vi "test-pose3d.vi"(8 "error in (no error)":errorcluster) -> (0 "error out":errorcluster, 3 "All PASSED":bool)   [LabVIEW 2019]
uses:
  <vilib>/Rock Robotics/WPI/ThirdParty/JAS_Junk/TrajLib/VI/Pose3d_getTranslation3d.vi
  <vilib>/Rock Robotics/WPI/ThirdParty/JAS_Junk/TrajLib/VI/Transform3d_GetTranslation3d.vi
  <vilib>/Rock Robotics/WPI/ThirdParty/JAS_Junk/TrajLib/VI/Translation3d_Plus.vi
  <vilib>/Rock Robotics/WPI/ThirdParty/JAS_Junk/TrajLib/VI/Translation3d_RotateBy.vi
  <vilib>/Rock Robotics/WPI/ThirdParty/JAS_Junk/TrajLib/VI/Rotation3d_Plus.vi
  <vilib>/Rock Robotics/WPI/ThirdParty/JAS_Junk/TrajLib/Rotation2d_CreateAngle.vi
  <vilib>/Rock Robotics/WPI/ThirdParty/JAS_Junk/TrajLib/Translation2d_Create.vi
  <vilib>/Rock Robotics/WPI/ThirdParty/JAS_Junk/TrajLib/VI/Translation3d_ToTranslation2d.vi
  <vilib>/Rock Robotics/WPI/ThirdParty/JAS_Junk/TrajLib/VI/Rotation3d_ToRotation2d.vi
  <vilib>/Rock Robotics/WPI/ThirdParty/JAS_Junk/TrajLib/Pose2d_New_TRRO.vi
  <vilib>/Rock Robotics/WPI/ThirdParty/JAS_Junk/TrajLib/Translation2d_Equals.vi
  <vilib>/Rock Robotics/WPI/ThirdParty/JAS_Junk/TrajLib/Rotation2d_Equals.vi
  <vilib>/Rock Robotics/WPI/ThirdParty/JAS_Junk/TrajLib/VI/Rotation3d_Create_Default.vi
  <vilib>/Rock Robotics/WPI/ThirdParty/JAS_Junk/TrajLib/VI/Vector_Norm.vi
  <vilib>/Rock Robotics/WPI/ThirdParty/JAS_Junk/TrajLib/VecBuilder_ArrayBy1Fill.vi
  <vilib>/Rock Robotics/WPI/ThirdParty/JAS_Junk/TrajLib/VI/Translation3d_GetXYZ.vi
  <vilib>/Rock Robotics/WPI/ThirdParty/JAS_Junk/TrajLib/VI/Translation3d_Equals.vi
  <vilib>/Rock Robotics/WPI/ThirdParty/JAS_Junk/TrajLib/VI/Rotation3d_Equals.vi
  <vilib>/Rock Robotics/WPI/ThirdParty/JAS_Junk/TrajLib/VI/Transform3d_Create_Pose3dPose3d.vi
  <vilib>/Rock Robotics/WPI/ThirdParty/JAS_Junk/TrajLib/VI/Quaternion_Times.vi
  <vilib>/Rock Robotics/WPI/ThirdParty/JAS_Junk/TrajLib/VI/Quaternion_Inverse.vi
  <vilib>/Rock Robotics/WPI/ThirdParty/JAS_Junk/TrajLib/VI/Rotation3d_RotateBy.vi
  <vilib>/Rock Robotics/WPI/ThirdParty/JAS_Junk/TrajLib/Util_CalcDist.vi
  <vilib>/Rock Robotics/WPI/ThirdParty/JAS_Junk/TrajLib/VI/Quaternion_New_Default.vi
  <vilib>/Rock Robotics/WPI/ThirdParty/JAS_Junk/TrajLib/MatBuilder_Create.vi
  <vilib>/Rock Robotics/WPI/ThirdParty/JAS_Junk/TrajLib/VI/Quaternion_Equals.vi
  <vilib>/Rock Robotics/WPI/ThirdParty/JAS_Junk/TrajLib/VI/Translation3d_Minus.vi
  <vilib>/Rock Robotics/WPI/ThirdParty/JAS_Junk/TrajLib/VI/Rotation3d_UnaryMinus.vi
  <vilib>/Rock Robotics/WPI/ThirdParty/JAS_Junk/TrajLib/VI/Rotation3d_Minus.vi
  <vilib>/Rock Robotics/WPI/ThirdParty/JAS_Junk/TrajLib/VI/Quaternion_Get_Vect.vi
  <vilib>/Rock Robotics/WPI/ThirdParty/JAS_Junk/TrajLib/VI/Quaternion_Get_W.vi
  <vilib>/Rock Robotics/WPI/ThirdParty/JAS_Junk/TrajLib/VI/Quaternion_Normalize.vi
  <vilib>/Rock Robotics/WPI/ThirdParty/JAS_Junk/TrajLib/Trajectory_Library.lvlib
panel:
  out "Exp/Log \nTest Passed":bool
  # "Pose 3D test"
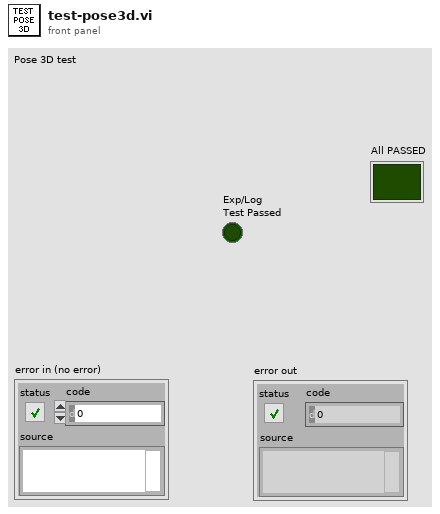
[diagram p1: front panel]
types:
  T1 = typedef "Trajectory_Library.lvlib/TRANSLATION3D.ctl" = cluster{"X":dbl, "Y":dbl, "Z":dbl}
  T2 = typedef "Trajectory_Library.lvlib/ROTATION3D.ctl" = cluster{"Q_quaternion":T3}
  T3 = typedef "Trajectory_Library.lvlib/QUATERNION.ctl" = cluster{"R":dbl, "V":dbl[]}
  T4 = typedef "Trajectory_Library.lvlib/POSE3D.ctl" = cluster{"Translation3d":T1, "Rotation3d":T2}
  T5 = typedef "Trajectory_Library.lvlib/TRANSFORM3D.ctl" = cluster{"TRANSLATION3D":T1, "ROTATION3D":T2, "XF":bool}
  T6 = typedef "Trajectory_Library.lvlib/POSE2D.ctl" = cluster{"TRANSLATION":T7, "ROTATION":T8}
  T7 = typedef "Trajectory_Library.lvlib/TRANSLATION2D.ctl" = cluster{"X":dbl, "Y":dbl}
  T8 = typedef "Trajectory_Library.lvlib/ROTATION2D.ctl" = cluster{"VALUE":dbl, "COS":dbl, "SIN":dbl}
  T9 = typedef "Trajectory_Library.lvlib/TWIST3D.ctl" = cluster{"dX":dbl, "dY":dbl, "dZ":dbl, "rX":dbl, "rY":dbl, "rZ":dbl}
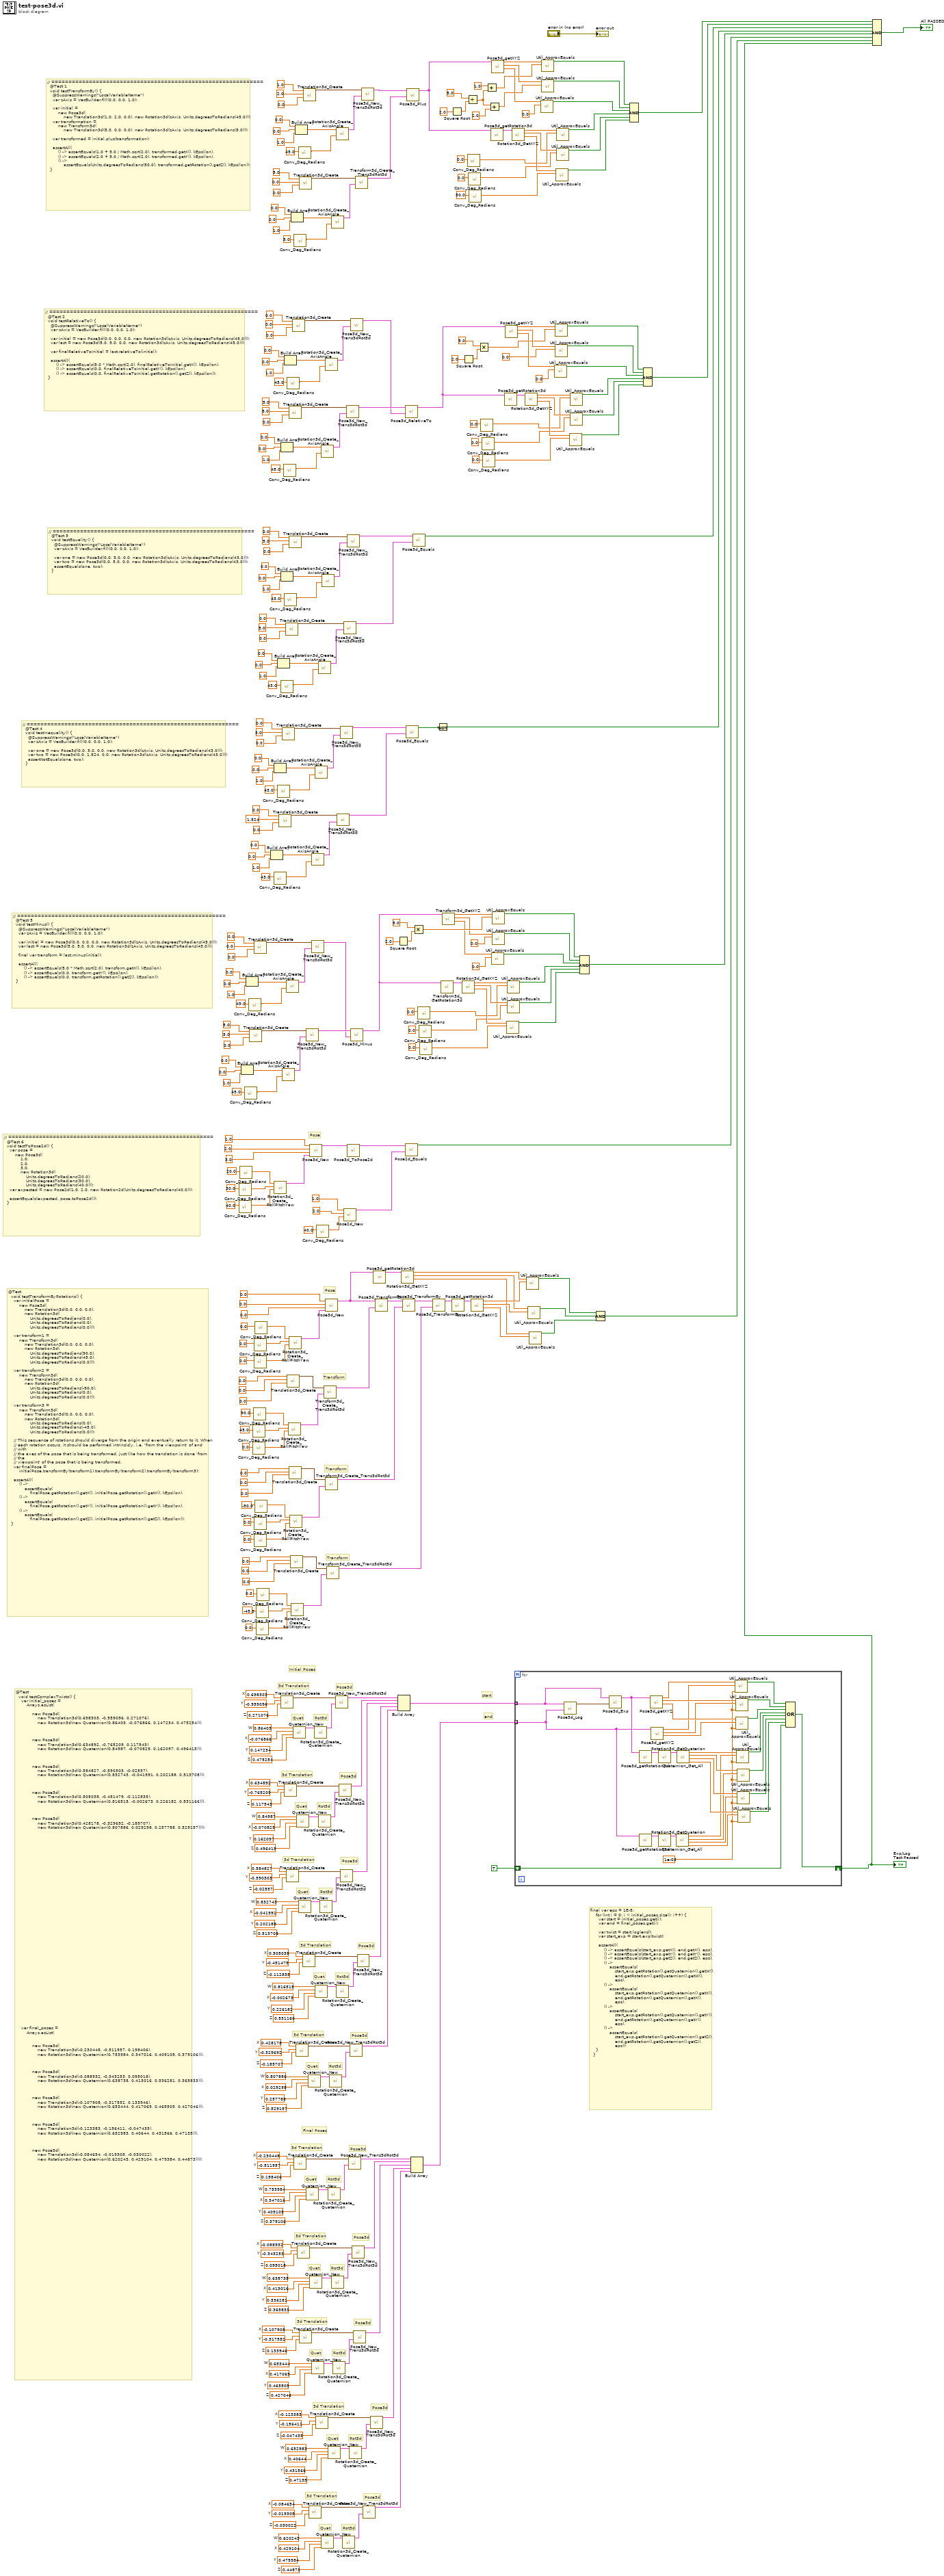
[diagram p0: block diagram]
diagram:
  w13 = 0.620243  # W
  w14 = 0.429104  # X
  w15 = 0.479384  # Y
  w16 = 0.44873  # Z
  w19 = -0.030022  # Z
  w18 = -0.084654  # X
  w17 = -0.019305  # Y
  w23 = 0.652983  # W
  w24 = 0.40644  # X
  w25 = 0.431566  # Y
  w26 = 0.47135  # Z
  w29 = -0.047435  # Z
  w28 = -0.123383  # X
  w27 = -0.156411  # Y
  w33 = 0.653444  # W
  w34 = 0.417069  # X
  w35 = 0.465505  # Y
  w36 = 0.427046  # Z
  w39 = 0.133946  # Z
  w38 = -0.107908  # X
  w37 = -0.317552  # Y
  w43 = 0.638738  # W
  w44 = 0.413016  # X
  w45 = 0.536281  # Y
  w46 = 0.365833  # Z
  w49 = 0.095018  # Z
  w48 = -0.088932  # X
  w47 = -0.343253  # Y
  w53 = 0.753984  # W
  w54 = 0.347016  # X
  w55 = 0.409105  # Y
  w56 = 0.379106  # Z
  w59 = 0.198406  # Z
  w58 = -0.230448  # X
  w57 = -0.511957  # Y
  w68 = 0.807886  # W
  w69 = 0.029298  # X
  w70 = 0.257788  # Y
  w71 = 0.529157  # Z
  w74 = -0.189707  # Z
  w73 = 0.428178  # X
  w72 = -0.329692  # Y
  w78 = 0.816515  # W
  w79 = -0.002673  # X
  w80 = 0.226182  # Y
  w81 = 0.531166  # Z
  w84 = -0.112835  # Z
  w83 = 0.505038  # X
  w82 = -0.451479  # Y
  w88 = 0.832743  # W
  w89 = -0.041991  # X
  w90 = 0.202188  # Y
  w91 = 0.513708  # Z
  w94 = -0.02557  # Z
  w93 = 0.584827  # X
  w92 = -0.590303  # Y
  w98 = 0.84987  # W
  w99 = -0.070829  # X
  w100 = 0.162097  # Y
  w101 = 0.496415  # Z
  w104 = 0.117543  # Z
  w103 = 0.634892  # X
  w102 = -0.765209  # Y
  w108 = 0.86403  # W
  w109 = -0.076866  # X
  w110 = 0.147234  # Y
  w111 = 0.475254  # Z
  w114 = 0.271076  # Z
  w113 = 0.698303  # X
  w112 = -0.959096  # Y
  # "end"
  # "start"
  # "final var eps = 1E-5;\n    for (int i = 0; i < initial_poses.size(); i++) {\n      var start = initial_poses.get(i);\n      var end = final_poses.get(i);\n\n      var twist = start.log(end);\n      var start_exp = start.exp(twist);\n\n      assertAll(\n          () -> assertEquals(start_exp.getX(), end.getX(), eps),\n          () -> assertEquals(start_exp.getY(), end.getY(), eps),\n          () -> assertEquals(start_exp.getZ(), end.getZ(), eps),\n          () ->\n              assertEquals(\n                  start_exp.getRotation().getQuaternion().getW(),\n                  end.getRotation().getQuaternion().getW(),\n                  eps),\n          () ->\n              assertEquals(\n                  start_exp.getRotation().getQuaternion().getX(),\n                  end.getRotation().getQuaternion().getX(),\n                  eps),\n          () ->\n              assertEquals(\n                  start_exp.getRotation().getQuaternion().getY(),\n                  end.getRotation().getQuaternion().getY(),\n                  eps),\n          () ->\n              assertEquals(\n                  start_exp.getRotation().getQuaternion().getZ(),\n                  end.getRotation().getQuaternion().getZ(),\n                  eps));\n    }\n  }"
  # "Rot3d"
  # "Pose3d"
  # "Quat"
  # "3d Translation"
  # "Rot3d"
  # "Pose3d"
  # "Quat"
  # "3d Translation"
  # "Rot3d"
  # "Pose3d"
  # "Quat"
  # "3d Translation"
  # "Rot3d"
  # "Pose3d"
  # "Quat"
  # "3d Translation"
  # "Final Poses"
  # "Rot3d"
  # "Pose3d"
  # "Quat"
  # "3d Translation"
  # "Rot3d"
  # "Pose3d"
  # "Quat"
  # "3d Translation"
  # "Rot3d"
  # "Pose3d"
  # "Quat"
  # "3d Translation"
  # "Rot3d"
  # "Pose3d"
  # "Quat"
  # "3d Translation"
  # "Rot3d"
  # "Pose3d"
  # "Quat"
  # "3d Translation"
  # "Initial Poses"
  # "Rot3d"
  # "Pose3d"
  # "Quat"
  # "3d Translation"
  # "@Test\n  void testComplexTwists() {\n    var initial_poses =\n        Arrays.asList(\n\n            new Pose3d(\n                new Translation3d(0.698303, -0.959096, 0.271076),\n                new Rotation3d(new Quaternion(0.86403, -0.076866, 0.147234, 0.475254))),\n\n\n\n            new Pose3d(\n                new Translation3d(0.634892, -0.765209, 0.117543),\n                new Rotation3d(new Quaternion(0.84987, -0.070829, 0.162097, 0.496415))),\n\n\n\n            new Pose3d(\n                new Translation3d(0.584827, -0.590303, -0.02557),\n                new Rotation3d(new Quaternion(0.832743, -0.041991, 0.202188, 0.513708))),\n\n\n\n            new Pose3d(\n                new Translation3d(0.505038, -0.451479, -0.112835),\n                new Rotation3d(new Quaternion(0.816515, -0.002673, 0.226182, 0.531166))),\n\n\n\n            new Pose3d(\n                new Translation3d(0.428178, -0.329692, -0.189707),\n                new Rotation3d(new Quaternion(0.807886, 0.029298, 0.257788, 0.529157))));\n\n\n\n\n\n\n\n\n\n\n\n\n\n\n\n\n\n\n\n\n\n\n\n\n\n\n\n\n\n\n\n\n\n\n\n\n\n\n\n\n\n\n\n\n\n    var final_poses =\n        Arrays.asList(\n\n\n            new Pose3d(\n                new Translation3d(-0.230448, -0.511957, 0.198406),\n                new Rotation3d(new Quaternion(0.753984, 0.347016, 0.409105, 0.379106))),\n\n\n\n            new Pose3d(\n                new Translation3d(-0.088932, -0.343253, 0.095018),\n                new Rotation3d(new Quaternion(0.638738, 0.413016, 0.536281, 0.365833))),\n\n\n\n            new Pose3d(\n                new Translation3d(-0.107908, -0.317552, 0.133946),\n                new Rotation3d(new Quaternion(0.653444, 0.417069, 0.465505, 0.427046))),\n\n\n\n            new Pose3d(\n                new Translation3d(-0.123383, -0.156411, -0.047435),\n                new Rotation3d(new Quaternion(0.652983, 0.40644, 0.431566, 0.47135))),\n\n\n\n            new Pose3d(\n                new Translation3d(-0.084654, -0.019305, -0.030022),\n                new Rotation3d(new Quaternion(0.620243, 0.429104, 0.479384, 0.44873))));"
  # "Transform"
  # "Transform"
  # "Transform"
  # "Pose"
  # "Pose"
  # "@Test\n  void testTransformByRotations() {\n    var initialPose =\n        new Pose3d(\n            new Translation3d(0.0, 0.0, 0.0),\n            new Rotation3d(\n                Units.degreesToRadians(0.0),\n                Units.degreesToRadians(0.0),\n                Units.degreesToRadians(0.0)));\n\n    var transform1 =\n        new Transform3d(\n            new Translation3d(0.0, 0.0, 0.0),\n            new Rotation3d(\n                Units.degreesToRadians(90.0),\n                Units.degreesToRadians(45.0),\n                Units.degreesToRadians(0.0)));\n\n    var transform2 =\n        new Transform3d(\n            new Translation3d(0.0, 0.0, 0.0),\n            new Rotation3d(\n                Units.degreesToRadians(-90.0),\n                Units.degreesToRadians(0.0),\n                Units.degreesToRadians(0.0)));\n\n    var transform3 =\n        new Transform3d(\n            new Translation3d(0.0, 0.0, 0.0),\n            new Rotation3d(\n                Units.degreesToRadians(0.0),\n                Units.degreesToRadians(-45.0),\n                Units.degreesToRadians(0.0)));\n\n    // This sequence of rotations should diverge from the origin and eventually return to it. When\n    // each rotation occurs, it should be performed intrinsicly, i.e. 'from the viewpoint' of and\n    // with\n    // the axes of the pose that is being transformed, just like how the translation is done 'from\n    // the\n    // viewpoint' of the pose that is being transformed.\n    var finalPose =\n        initialPose.transformBy(transform1).transformBy(transform2).transformBy(transform3);\n\n    assertAll(\n        () ->\n            assertEquals(\n                finalPose.getRotation().getX(), initialPose.getRotation().getX(), kEpsilon),\n        () ->\n            assertEquals(\n                finalPose.getRotation().getY(), initialPose.getRotation().getY(), kEpsilon),\n        () ->\n            assertEquals(\n                finalPose.getRotation().getZ(), initialPose.getRotation().getZ(), kEpsilon));\n  }"
  # "// ============================================================\n  @Test 6\n  void testToPose2d() {\n    var pose =\n        new Pose3d(\n            1.0,\n            2.0,\n            3.0,\n            new Rotation3d(\n                Units.degreesToRadians(20.0),\n                Units.degreesToRadians(30.0),\n                Units.degreesToRadians(40.0)));\n    var expected = new Pose2d(1.0, 2.0, new Rotation2d(Units.degreesToRadians(40.0)));\n\n    assertEquals(expected, pose.toPose2d());\n  }"
  # "// =============================================================\n  @Test 5\n  void testMinus() {\n    @SuppressWarnings(\"LocalVariableName\")\n    var zAxis = VecBuilder.fill(0.0, 0.0, 1.0);\n\n    var initial = new Pose3d(0.0, 0.0, 0.0, new Rotation3d(zAxis, Units.degreesToRadians(45.0)));\n    var last = new Pose3d(5.0, 5.0, 0.0, new Rotation3d(zAxis, Units.degreesToRadians(45.0)));\n\n    final var transform = last.minus(initial);\n\n    assertAll(\n        () -> assertEquals(5.0 * Math.sqrt(2.0), transform.getX(), kEpsilon),\n        () -> assertEquals(0.0, transform.getY(), kEpsilon),\n        () -> assertEquals(0.0, transform.getRotation().getZ(), kEpsilon));\n  }"
  # "// ==============================================================\n  @Test 4\n  void testInequality() {\n    @SuppressWarnings(\"LocalVariableName\")\n    var zAxis = VecBuilder.fill(0.0, 0.0, 1.0);\n\n    var one = new Pose3d(0.0, 5.0, 0.0, new Rotation3d(zAxis, Units.degreesToRadians(43.0)));\n    var two = new Pose3d(0.0, 1.524, 0.0, new Rotation3d(zAxis, Units.degreesToRadians(43.0)));\n    assertNotEquals(one, two);\n  }"
  # "// ===========================================================\n  @Test 3\n  void testEquality() {\n    @SuppressWarnings(\"LocalVariableName\")\n    var zAxis = VecBuilder.fill(0.0, 0.0, 1.0);\n\n    var one = new Pose3d(0.0, 5.0, 0.0, new Rotation3d(zAxis, Units.degreesToRadians(43.0)));\n    var two = new Pose3d(0.0, 5.0, 0.0, new Rotation3d(zAxis, Units.degreesToRadians(43.0)));\n    assertEquals(one, two);\n  }"
  # "// =============================================================\n  @Test 2\n  void testRelativeTo() {\n    @SuppressWarnings(\"LocalVariableName\")\n    var zAxis = VecBuilder.fill(0.0, 0.0, 1.0);\n\n    var initial = new Pose3d(0.0, 0.0, 0.0, new Rotation3d(zAxis, Units.degreesToRadians(45.0)));\n    var last = new Pose3d(5.0, 5.0, 0.0, new Rotation3d(zAxis, Units.degreesToRadians(45.0)));\n\n    var finalRelativeToInitial = last.relativeTo(initial);\n\n    assertAll(\n        () -> assertEquals(5.0 * Math.sqrt(2.0), finalRelativeToInitial.getX(), kEpsilon),\n        () -> assertEquals(0.0, finalRelativeToInitial.getY(), kEpsilon),\n        () -> assertEquals(0.0, finalRelativeToInitial.getRotation().getZ(), kEpsilon));\n  }"
  # "// ==============================================================\n  @Test 1\n  void testTransformBy() {\n    @SuppressWarnings(\"LocalVariableName\")\n    var zAxis = VecBuilder.fill(0.0, 0.0, 1.0);\n\n    var initial =\n        new Pose3d(\n            new Translation3d(1.0, 2.0, 0.0), new Rotation3d(zAxis, Units.degreesToRadians(45.0)));\n    var transformation =\n        new Transform3d(\n            new Translation3d(5.0, 0.0, 0.0), new Rotation3d(zAxis, Units.degreesToRadians(5.0)));\n\n    var transformed = initial.plus(transformation);\n\n    assertAll(\n        () -> assertEquals(1.0 + 5.0 / Math.sqrt(2.0), transformed.getX(), kEpsilon),\n        () -> assertEquals(2.0 + 5.0 / Math.sqrt(2.0), transformed.getY(), kEpsilon),\n        () ->\n            assertEquals(Units.degreesToRadians(50.0), transformed.getRotation().getZ(), kEpsilon));\n  }"
  n1 = call <vilib>:"Conv_Deg_Radians.vi"("Degress"=30.0) -> ("Radians"=w187:dbl)  [unwired: 10 in]
  n2 = call <vilib>:"Conv_Deg_Radians.vi"("Degress"=40.0) -> ("Radians"=w186:dbl)  [unwired: 10 in]
  n3 = call <vilib>:"Conv_Deg_Radians.vi"("Degress"=20.0) -> ("Radians"=w188:dbl)  [unwired: 10 in]
  n4 = Build Array(0.0 ("element"), 0.0 ("element"), 1.0 ("element")) -> (w234:dbl[])
  n5 = call <vilib>:"Conv_Deg_Radians.vi"("Degress"=45.0) -> ("Radians"=w232:dbl)  [unwired: 10 in]
  n6 = Build Array(0.0 ("element"), 0.0 ("element"), 1.0 ("element")) -> (w245:dbl[])
  n7 = call <vilib>:"Conv_Deg_Radians.vi"("Degress"=45.0) -> ("Radians"=w243:dbl)  [unwired: 10 in]
  n8 = call <vilib>:"Translation3d_Create.vi"("Z"=0.0, "Y"=5.0, "X"=5.0) -> ("TRANSLATION3D"=w225:T1)  [unwired: 8 in]
  n9 = call <vilib>:"Conv_Deg_Radians.vi"("Degress"=45.0) -> ("Radians"=w162:dbl)  [unwired: 10 in]
  n10 = call <vilib>:"Conv_Deg_Radians.vi"("Degress"=0.0) -> ("Radians"=w161:dbl)  [unwired: 10 in]
  n11 = call <vilib>:"Conv_Deg_Radians.vi"("Degress"=90.0) -> ("Radians"=w163:dbl)  [unwired: 10 in]
  n12 = call <vilib>:"Translation3d_Create.vi"("Z"=0.0, "Y"=0.0, "X"=0.0) -> ("TRANSLATION3D"=w236:T1)  [unwired: 8 in]
  n13 = call <vilib>:"Conv_Deg_Radians.vi"("Degress"=0.0) -> ("Radians"=w169:dbl)  [unwired: 10 in]
  n14 = call <vilib>:"Conv_Deg_Radians.vi"("Degress"=0.0) -> ("Radians"=w168:dbl)  [unwired: 10 in]
  n15 = call <vilib>:"Conv_Deg_Radians.vi"("Degress"=0.0) -> ("Radians"=w151:dbl)  [unwired: 10 in]
  n16 = call <vilib>:"Conv_Deg_Radians.vi"("Degress"=0.0) -> ("Radians"=w150:dbl)  [unwired: 10 in]
  n17 = call <vilib>:"Conv_Deg_Radians.vi"("Degress"=0.0) -> ("Radians"=w170:dbl)  [unwired: 10 in]
  n18 = call <vilib>:"Conv_Deg_Radians.vi"("Degress"=-90.0) -> ("Radians"=w152:dbl)  [unwired: 10 in]
  n19 = call <vilib>:"Conv_Deg_Radians.vi"("Degress"=-45.0) -> ("Radians"=w140:dbl)  [unwired: 10 in]
  n20 = call <vilib>:"Conv_Deg_Radians.vi"("Degress"=0.0) -> ("Radians"=w139:dbl)  [unwired: 10 in]
  n21 = call <vilib>:"Conv_Deg_Radians.vi"("Degress"=0.0) -> ("Radians"=w141:dbl)  [unwired: 10 in]
  n22 = Build Array(0.0 ("element"), 0.0 ("element"), 1.0 ("element")) -> (w260:dbl[])
  n23 = call <vilib>:"Conv_Deg_Radians.vi"("Degress"=43.0) -> ("Radians"=w258:dbl)  [unwired: 10 in]
  n24 = Build Array(0.0 ("element"), 0.0 ("element"), 1.0 ("element")) -> (w271:dbl[])
  n25 = call <vilib>:"Rotation3d_Create_RollPitchYaw.vi"("Yaw"=w186, "Pitch"=w187, "Roll"=w188) -> ("Rotation3d"=w185:T2)  [unwired: 8 in]
  n26 = Build Array(0.0 ("element"), 0.0 ("element"), 1.0 ("element")) -> (w285:dbl[])
  n27 = call <vilib>:"Conv_Deg_Radians.vi"("Degress"=43.0) -> ("Radians"=w269:dbl)  [unwired: 10 in]
  n28 = call <vilib>:"Translation3d_Create.vi"("Z"=0.0, "Y"=1.524, "X"=0.0) -> ("TRANSLATION3D"=w251:T1)  [unwired: 8 in]
  n29 = Build Array(0.0 ("element"), 0.0 ("element"), 1.0 ("element")) -> (w336:dbl[])
  n30 = call <vilib>:"Conv_Deg_Radians.vi"("Degress"=43.0) -> ("Radians"=w283:dbl)  [unwired: 10 in]
  n31 = Build Array(0.0 ("element"), 0.0 ("element"), 1.0 ("element")) -> (w296:dbl[])
  n32 = call <vilib>:"Translation3d_Create.vi"("Z"=w114, "Y"=w112, "X"=w113) -> ("TRANSLATION3D"=w107:T1)  [unwired: 8 in]
  n33 = call <vilib>:"Rotation3d_Create_AxisAngle.vi"("Angle"=w232, "Axis Vector"=w234) -> ("Rotation3d"=w224:T2)  [unwired: 9 in]
  n34 = call <vilib>:"Translation3d_Create.vi"("Z"=0.0, "Y"=5.0, "X"=0.0) -> ("TRANSLATION3D"=w262:T1)  [unwired: 8 in]
  n35 = call <vilib>:"Conv_Deg_Radians.vi"("Degress"=45.0) -> ("Radians"=w334:dbl)  [unwired: 10 in]
  n36 = Build Array(0.0 ("element"), 0.0 ("element"), 1.0 ("element")) -> (w347:dbl[])
  n37 = call <vilib>:"Conv_Deg_Radians.vi"("Degress"=43.0) -> ("Radians"=w294:dbl)  [unwired: 10 in]
  n38 = call <vilib>:"Translation3d_Create.vi"("Z"=w104, "Y"=w102, "X"=w103) -> ("TRANSLATION3D"=w97:T1)  [unwired: 8 in]
  n39 = call <vilib>:"Translation3d_Create.vi"("Z"=0.0, "Y"=5.0, "X"=0.0) -> ("TRANSLATION3D"=w276:T1)  [unwired: 8 in]
  n40 = call <vilib>:"Translation3d_Create.vi"("Z"=w94, "Y"=w92, "X"=w93) -> ("TRANSLATION3D"=w87:T1)  [unwired: 8 in]
  n41 = call <vilib>:"Rotation3d_Create_AxisAngle.vi"("Angle"=w243, "Axis Vector"=w245) -> ("Rotation3d"=w235:T2)  [unwired: 9 in]
  n42 = call <vilib>:"Conv_Deg_Radians.vi"("Degress"=45.0) -> ("Radians"=w345:dbl)  [unwired: 10 in]
  n43 = call <vilib>:"Translation3d_Create.vi"("Z"=0.0, "Y"=0.0, "X"=0.0) -> ("TRANSLATION3D"=w159:T1)  [unwired: 8 in]
  n44 = call <vilib>:"Rotation3d_Create_RollPitchYaw.vi"("Yaw"=w161, "Pitch"=w162, "Roll"=w163) -> ("Rotation3d"=w160:T2)  [unwired: 8 in]
  n45 = call <vilib>:"Translation3d_Create.vi"("Z"=0.0, "Y"=5.0, "X"=5.0) -> ("TRANSLATION3D"=w327:T1)  [unwired: 8 in]
  n46 = call <vilib>:"Translation3d_Create.vi"("Z"=0.0, "Y"=0.0, "X"=0.0) -> ("TRANSLATION3D"=w148:T1)  [unwired: 8 in]
  n47 = call <vilib>:"Translation3d_Create.vi"("Z"=0.0, "Y"=5.0, "X"=0.0) -> ("TRANSLATION3D"=w287:T1)  [unwired: 8 in]
  n48 = call <vilib>:"Rotation3d_Create_RollPitchYaw.vi"("Yaw"=w168, "Pitch"=w169, "Roll"=w170) -> ("Rotation3d"=w167:T2)  [unwired: 8 in]
  n49 = call <vilib>:"Rotation3d_Create_RollPitchYaw.vi"("Yaw"=w150, "Pitch"=w151, "Roll"=w152) -> ("Rotation3d"=w149:T2)  [unwired: 8 in]
  n50 = call <vilib>:"Translation3d_Create.vi"("Z"=0.0, "Y"=0.0, "X"=0.0) -> ("TRANSLATION3D"=w137:T1)  [unwired: 8 in]
  n51 = Build Array(0.0 ("element"), 0.0 ("element"), 1.0 ("element")) -> (w391:dbl[])
  n52 = call <vilib>:"Rotation3d_Create_RollPitchYaw.vi"("Yaw"=w139, "Pitch"=w140, "Roll"=w141) -> ("Rotation3d"=w138:T2)  [unwired: 8 in]
  n53 = call <vilib>:"Translation3d_Create.vi"("Z"=0.0, "Y"=0.0, "X"=0.0) -> ("TRANSLATION3D"=w338:T1)  [unwired: 8 in]
  n54 = call <vilib>:"Quaternion_New.vi"("Z"=w111, "Y"=w110, "X"=w109, "W"=w108) -> ("out Quaternion"=w106:T3)  [unwired: 7 in]
  n55 = call <vilib>:"Conv_Deg_Radians.vi"("Degress"=5.0) -> ("Radians"=w389:dbl)  [unwired: 10 in]
  n56 = call <vilib>:"Translation3d_Create.vi"("Z"=w59, "Y"=w57, "X"=w58) -> ("TRANSLATION3D"=w52:T1)  [unwired: 8 in]
  n57 = Build Array(0.0 ("element"), 0.0 ("element"), 1.0 ("element")) -> (w402:dbl[])
  n58 = call <vilib>:"Translation3d_Create.vi"("Z"=w74, "Y"=w72, "X"=w73) -> ("TRANSLATION3D"=w67:T1)  [unwired: 8 in]
  n59 = call <vilib>:"Quaternion_New.vi"("Z"=w101, "Y"=w100, "X"=w99, "W"=w98) -> ("out Quaternion"=w96:T3)  [unwired: 7 in]
  n60 = call <vilib>:"Translation3d_Create.vi"("Z"=w49, "Y"=w47, "X"=w48) -> ("TRANSLATION3D"=w42:T1)  [unwired: 8 in]
  n61 = call <vilib>:"Conv_Deg_Radians.vi"("Degress"=45.0) -> ("Radians"=w400:dbl)  [unwired: 10 in]
  n62 = call <vilib>:"Quaternion_New.vi"("Z"=w91, "Y"=w90, "X"=w89, "W"=w88) -> ("out Quaternion"=w86:T3)  [unwired: 7 in]
  n63 = call <vilib>:"Translation3d_Create.vi"("Z"=0.0, "Y"=0.0, "X"=5.0) -> ("TRANSLATION3D"=w382:T1)  [unwired: 8 in]
  n64 = call <vilib>:"Translation3d_Create.vi"("Z"=w39, "Y"=w37, "X"=w38) -> ("TRANSLATION3D"=w32:T1)  [unwired: 8 in]
  n65 = call <vilib>:"Translation3d_Create.vi"("Z"=w84, "Y"=w82, "X"=w83) -> ("TRANSLATION3D"=w77:T1)  [unwired: 8 in]
  n66 = call <vilib>:"Translation3d_Create.vi"("Z"=0.0, "Y"=2.0, "X"=1.0) -> ("TRANSLATION3D"=w393:T1)  [unwired: 8 in]
  n67 = call <vilib>:"Pose3d_New_Trans3dRot3d.vi"("Rotation3d"=w224, "Translation3d"=w225) -> ("outPose3d"=w197:T4)  [unwired: 9 in]
  n68 = call <vilib>:"Quaternion_New.vi"("Z"=w56, "Y"=w55, "X"=w54, "W"=w53) -> ("out Quaternion"=w51:T3)  [unwired: 7 in]
  n69 = call <vilib>:"Quaternion_New.vi"("Z"=w71, "Y"=w70, "X"=w69, "W"=w68) -> ("out Quaternion"=w66:T3)  [unwired: 7 in]
  n70 = call <vilib>:"Translation3d_Create.vi"("Z"=w19, "Y"=w17, "X"=w18) -> ("TRANSLATION3D"=w12:T1)  [unwired: 8 in]
  n71 = call <vilib>:"Pose3d_New.vi"("Rotation3d"=w185, "z"=3.0 ("Z"), "Y"=2.0, "X"=1.0) -> ("out Pose3d"=w184:T4)  [unwired: 7 in]
  n72 = call <vilib>:"Quaternion_New.vi"("Z"=w46, "Y"=w45, "X"=w44, "W"=w43) -> ("out Quaternion"=w41:T3)  [unwired: 7 in]
  n73 = call <vilib>:"Rotation3d_Create_AxisAngle.vi"("Angle"=w258, "Axis Vector"=w260) -> ("Rotation3d"=w250:T2)  [unwired: 9 in]
  n74 = call <vilib>:"Quaternion_New.vi"("Z"=w36, "Y"=w35, "X"=w34, "W"=w33) -> ("out Quaternion"=w31:T3)  [unwired: 7 in]
  n75 = call <vilib>:"Pose3d_New_Trans3dRot3d.vi"("Rotation3d"=w235, "Translation3d"=w236) -> ("outPose3d"=w196:T4)  [unwired: 9 in]
  n76 = call <vilib>:"Rotation3d_Create_Quaternion.vi"("Quaternion"=w106) -> ("Rotation3d"=w105:T2)  [unwired: 10 in]
  n77 = call <vilib>:"Rotation3d_Create_AxisAngle.vi"("Angle"=w269, "Axis Vector"=w271) -> ("Rotation3d"=w261:T2)  [unwired: 9 in]
  n78 = call <vilib>:"Quaternion_New.vi"("Z"=w81, "Y"=w80, "X"=w79, "W"=w78) -> ("out Quaternion"=w76:T3)  [unwired: 7 in]
  n79 = call <vilib>:"Translation3d_Create.vi"("Z"=w29, "Y"=w27, "X"=w28) -> ("TRANSLATION3D"=w22:T1)  [unwired: 8 in]
  n80 = call <vilib>:"Conv_Deg_Radians.vi"("Degress"=40.0) -> ("Radians"=w180:dbl)  [unwired: 10 in]
  n81 = call <vilib>:"Rotation3d_Create_AxisAngle.vi"("Angle"=w283, "Axis Vector"=w285) -> ("Rotation3d"=w275:T2)  [unwired: 9 in]
  n82 = call <vilib>:"Rotation3d_Create_Quaternion.vi"("Quaternion"=w96) -> ("Rotation3d"=w95:T2)  [unwired: 10 in]
  n83 = call <vilib>:"Rotation3d_Create_Quaternion.vi"("Quaternion"=w86) -> ("Rotation3d"=w85:T2)  [unwired: 10 in]
  n84 = call <vilib>:"Quaternion_New.vi"("Z"=w16, "Y"=w15, "X"=w14, "W"=w13) -> ("out Quaternion"=w11:T3)  [unwired: 7 in]
  n85 = call <vilib>:"Rotation3d_Create_AxisAngle.vi"("Angle"=w334, "Axis Vector"=w336) -> ("Rotation3d"=w326:T2)  [unwired: 9 in]
  n86 = call <vilib>:"Rotation3d_Create_AxisAngle.vi"("Angle"=w294, "Axis Vector"=w296) -> ("Rotation3d"=w286:T2)  [unwired: 9 in]
  n87 = call <vilib>:"Transform3d_Create_Trans3dRot3d.vi"("Rotation3d"=w160, "Translation3d"=w159) -> ("Transform3d"=w133:T5)  [unwired: 9 in]
  n88 = call <vilib>:"Rotation3d_Create_AxisAngle.vi"("Angle"=w345, "Axis Vector"=w347) -> ("Rotation3d"=w337:T2)  [unwired: 9 in]
  n89 = call <vilib>:"Pose3d_New.vi"("Rotation3d"=w167, "z"=0.0 ("Z"), "Y"=0.0, "X"=0.0) -> ("out Pose3d"=w128:T4)  [unwired: 7 in]
  n90 = call <vilib>:"Transform3d_Create_Trans3dRot3d.vi"("Rotation3d"=w149, "Translation3d"=w148) -> ("Transform3d"=w131:T5)  [unwired: 9 in]
  n91 = call <vilib>:"Transform3d_Create_Trans3dRot3d.vi"("Rotation3d"=w138, "Translation3d"=w137) -> ("Transform3d"=w129:T5)  [unwired: 9 in]
  n92 = call <vilib>:"Rotation3d_Create_Quaternion.vi"("Quaternion"=w51) -> ("Rotation3d"=w50:T2)  [unwired: 10 in]
  n93 = call <vilib>:"Quaternion_New.vi"("Z"=w26, "Y"=w25, "X"=w24, "W"=w23) -> ("out Quaternion"=w21:T3)  [unwired: 7 in]
  n94 = call <vilib>:"Rotation3d_Create_Quaternion.vi"("Quaternion"=w66) -> ("Rotation3d"=w65:T2)  [unwired: 10 in]
  n95 = call <vilib>:"Rotation3d_Create_Quaternion.vi"("Quaternion"=w41) -> ("Rotation3d"=w40:T2)  [unwired: 10 in]
  n96 = call <vilib>:"Rotation3d_Create_AxisAngle.vi"("Angle"=w389, "Axis Vector"=w391) -> ("Rotation3d"=w381:T2)  [unwired: 9 in]
  n97 = call <vilib>:"Rotation3d_Create_Quaternion.vi"("Quaternion"=w31) -> ("Rotation3d"=w30:T2)  [unwired: 10 in]
  n98 = call <vilib>:"Pose3d_New_Trans3dRot3d.vi"("Rotation3d"=w105, "Translation3d"=w107) -> ("outPose3d"=w64:T4)  [unwired: 9 in]
  n99 = call <vilib>:"Rotation3d_Create_AxisAngle.vi"("Angle"=w400, "Axis Vector"=w402) -> ("Rotation3d"=w392:T2)  [unwired: 9 in]
  n100 = call <vilib>:"Rotation3d_Create_Quaternion.vi"("Quaternion"=w76) -> ("Rotation3d"=w75:T2)  [unwired: 10 in]
  n101 = call <vilib>:"Pose3d_New_Trans3dRot3d.vi"("Rotation3d"=w250, "Translation3d"=w251) -> ("outPose3d"=w248:T4)  [unwired: 9 in]
  n102 = call <vilib>:"Pose3d_New_Trans3dRot3d.vi"("Rotation3d"=w95, "Translation3d"=w97) -> ("outPose3d"=w63:T4)  [unwired: 9 in]
  n103 = call <vilib>:"Pose3d_New_Trans3dRot3d.vi"("Rotation3d"=w261, "Translation3d"=w262) -> ("outPose3d"=w249:T4)  [unwired: 9 in]
  n104 = call <vilib>:"Pose3d_New_Trans3dRot3d.vi"("Rotation3d"=w85, "Translation3d"=w87) -> ("outPose3d"=w62:T4)  [unwired: 9 in]
  n105 = call <vilib>:"Rotation3d_Create_Quaternion.vi"("Quaternion"=w11) -> ("Rotation3d"=w10:T2)  [unwired: 10 in]
  n106 = call <vilib>:"Pose3d_New_Trans3dRot3d.vi"("Rotation3d"=w275, "Translation3d"=w276) -> ("outPose3d"=w273:T4)  [unwired: 9 in]
  n107 = call <vilib>:"Pose2d_New.vi"("Heading"=w180, "Y"=2.0 ("X"), "X"=1.0) -> ("out POSe"=w178:T6)  [unwired: 8 in]
  n108 = call <vilib>:"Pose3d_New_Trans3dRot3d.vi"("Rotation3d"=w326, "Translation3d"=w327) -> ("outPose3d"=w325:T4)  [unwired: 9 in]
  n109 = call <vilib>:"Pose3d_New_Trans3dRot3d.vi"("Rotation3d"=w286, "Translation3d"=w287) -> ("outPose3d"=w274:T4)  [unwired: 9 in]
  n110 = call <vilib>:"Pose3d_ToPose2d.vi"("in Pose3d"=w184) -> ("out Pose2d"=w179:T6)  [unwired: 10 in]
  n111 = call <vilib>:"Pose3d_New_Trans3dRot3d.vi"("Rotation3d"=w50, "Translation3d"=w52) -> ("outPose3d"=w9:T4)  [unwired: 9 in]
  n112 = call <vilib>:"Rotation3d_Create_Quaternion.vi"("Quaternion"=w21) -> ("Rotation3d"=w20:T2)  [unwired: 10 in]
  n113 = call <vilib>:"Pose3d_New_Trans3dRot3d.vi"("Rotation3d"=w65, "Translation3d"=w67) -> ("outPose3d"=w60:T4)  [unwired: 9 in]
  n114 = call <vilib>:"Pose3d_New_Trans3dRot3d.vi"("Rotation3d"=w337, "Translation3d"=w338) -> ("outPose3d"=w324:T4)  [unwired: 9 in]
  n115 = call <vilib>:"Pose3d_Minus.vi"("other Pose3d"=w196, "in Pose3d"=w197) -> ("outTransform3d"=w212:T5)  [unwired: 9 in]
  n116 = call <vilib>:"Pose3d_New_Trans3dRot3d.vi"("Rotation3d"=w40, "Translation3d"=w42) -> ("outPose3d"=w8:T4)  [unwired: 9 in]
  n117 = call <vilib>:"Pose3d_New_Trans3dRot3d.vi"("Rotation3d"=w30, "Translation3d"=w32) -> ("outPose3d"=w7:T4)  [unwired: 9 in]
  n118 = call <vilib>:"Transform3d_Create_Trans3dRot3d.vi"("Rotation3d"=w381, "Translation3d"=w382) -> ("Transform3d"=w366:T5)  [unwired: 9 in]
  n119 = call <vilib>:"Pose3d_New_Trans3dRot3d.vi"("Rotation3d"=w75, "Translation3d"=w77) -> ("outPose3d"=w61:T4)  [unwired: 9 in]
  n120 = call <vilib>:"Pose3d_New_Trans3dRot3d.vi"("Rotation3d"=w392, "Translation3d"=w393) -> ("outPose3d"=w367:T4)  [unwired: 9 in]
  n121 = call <vilib>:"Pose3d_New_Trans3dRot3d.vi"("Rotation3d"=w10, "Translation3d"=w12) -> ("outPose3d"=w5:T4)  [unwired: 9 in]
  n122 = call <vilib>:"Pose3d_New_Trans3dRot3d.vi"("Rotation3d"=w20, "Translation3d"=w22) -> ("outPose3d"=w6:T4)  [unwired: 9 in]
  n123 = call <vilib>:"Pose3d_getRotation3d.vi"("in Pose3d"=w128) -> ("out Rotation3d"=w127:T2)  [unwired: 10 in]
  n124 = call <vilib>:"Pose3d_TransformBy.vi"("other Transform3d"=w133, "in Pose3d"=w128) -> ("out POSE3d"=w132:T4)  [unwired: 9 in]
  n125 = Square Root(x=2.0) -> (sqrt(x)=w209:dbl)
  n126 = Build Array(w64, w63, w62, w61, w60) -> (w4:T4[])
  n127 = call <vilib>:"Rotation3d_GetXYZ.vi"("in Rotation3d"=w127) -> ("Z"=w120:dbl, "Y"=w122:dbl, "X"=w124:dbl)  [unwired: 8 in]
  n128 = call <vilib>:"Pose3d_TransformBy.vi"("other Transform3d"=w131, "in Pose3d"=w132) -> ("out POSE3d"=w130:T4)  [unwired: 9 in]
  n129 = call <vilib>:"Pose3d_RelativeTo.vi"("other Pose3d"=w324, "in Pose3d"=w325) -> ("out Pose3d"=w300:T4)  [unwired: 9 in]
  n130 = call <vilib>:"Pose2d_Equals.vi"("other POSE"=w178, "in POSE"=w179) -> ("Equals"=w177:bool)  [unwired: 9 in]
  n131 = call <vilib>:"Pose3d_Equals.vi"("other Pose3d"=w248, "in Pose3d"=w249) -> ("Equals"=w247:bool)  [unwired: 9 in]
  n132 = call <vilib>:"Pose3d_Plus.vi"("other Transform3d"=w366, "in Pose3d"=w367) -> ("out Pose3d"=w365:T4)  [unwired: 9 in]
  n133 = Build Array(w9, w8, w7, w6, w5) -> (w3:T4[])
  n134 = call <vilib>:"Pose3d_Equals.vi"("other Pose3d"=w273, "in Pose3d"=w274) -> ("Equals"=w272:bool)  [unwired: 9 in]
  n135 = Multiply(x=5.0, y=w209) -> (x*y=w201:dbl)
  n136 = call <vilib>:"Conv_Deg_Radians.vi"("Degress"=0.0) -> ("Radians"=w202:dbl)  [unwired: 10 in]
  n137 = call <vilib>:"Conv_Deg_Radians.vi"("Degress"=0.0) -> ("Radians"=w203:dbl)  [unwired: 10 in]
  n138 = call <vilib>:"Conv_Deg_Radians.vi"("Degress"=0.0) -> ("Radians"=w204:dbl)  [unwired: 10 in]
  n139 = call <vilib>:"Pose3d_TransformBy.vi"("other Transform3d"=w129, "in Pose3d"=w130) -> ("out POSE3d"=w126:T4)  [unwired: 9 in]
  n140 = Not(x=w247) -> (.not. x?=w246:bool)
  n141 = call <vilib>:"Transform3d_GetRotation3d.vi"("in Transform3d"=w212) -> ("Rotation3d"=w222:T2)  [unwired: 10 in]
  n142 = call <vilib>:"Transform3d_GetXYZ.vi"("inTransform3d"=w212) -> ("Z"=w198:dbl, "Y"=w199:dbl, "X"=w223:dbl)  [unwired: 8 in]
  n143 = Square Root(x=2.0) -> (sqrt(x)=w362:dbl)
  n144 = call <vilib>:"Pose3d_getRotation3d.vi"("in Pose3d"=w126) -> ("out Rotation3d"=w125:T2)  [unwired: 10 in]
  n145 = call <vilib>:"Rotation3d_GetXYZ.vi"("in Rotation3d"=w222) -> ("Z"=w219:dbl, "Y"=w220:dbl, "X"=w221:dbl)  [unwired: 8 in]
  n146 = Square Root(x=2.0) -> (sqrt(x)=w308:dbl)
  n147 = Divide(x=5.0, y=w362) -> (x/y=w359:dbl)
  n148 = call <vilib>:"Conv_Deg_Radians.vi"("Degress"=0.0) -> ("Radians"=w350:dbl)  [unwired: 10 in]
  n149 = call <vilib>:"Conv_Deg_Radians.vi"("Degress"=0.0) -> ("Radians"=w351:dbl)  [unwired: 10 in]
  n150 = call <vilib>:"Conv_Deg_Radians.vi"("Degress"=50.0) -> ("Radians"=w352:dbl)  [unwired: 10 in]
  n151 = call <vilib>:"Rotation3d_GetXYZ.vi"("in Rotation3d"=w125) -> ("Z"=w119:dbl, "Y"=w121:dbl, "X"=w123:dbl)  [unwired: 8 in]
  n152 = Multiply(x=5.0, y=w308) -> (x*y=w299:dbl)
  n153 = call <vilib>:"Conv_Deg_Radians.vi"("Degress"=0.0) -> ("Radians"=w301:dbl)  [unwired: 10 in]
  n154 = call <vilib>:"Conv_Deg_Radians.vi"("Degress"=0.0) -> ("Radians"=w302:dbl)  [unwired: 10 in]
  n155 = call <vilib>:"Conv_Deg_Radians.vi"("Degress"=0.0) -> ("Radians"=w303:dbl)  [unwired: 10 in]
  n156 = Add(x=1.0, y=w359) -> (x+y=w361:dbl)
  n157 = Add(x=w359, y=2.0) -> (x+y=w360:dbl)
  n158 = call <vilib>:"Pose3d_getRotation3d.vi"("in Pose3d"=w365) -> ("out Rotation3d"=w377:T2)  [unwired: 10 in]
  n159 = call <vilib>:"Util_ApproxEquals.vi"("Value 2"=0.0, "Value 1"=w198) -> ("ApproxEquals"=w216:bool)  [unwired: 9 in]
  n160 = call <vilib>:"Pose3d_getXYZ.vi"("in Pose3d"=w365) -> ("Z"=w378:dbl, "Y"=w379:dbl, "X"=w380:dbl)  [unwired: 8 in]
  n161 = call <vilib>:"Util_ApproxEquals.vi"("Value 2"=w201, "Value 1"=w223) -> ("ApproxEquals"=w218:bool)  [unwired: 9 in]
  n162 = call <vilib>:"Util_ApproxEquals.vi"("Value 2"=0.0, "Value 1"=w199) -> ("ApproxEquals"=w217:bool)  [unwired: 9 in]
  n163 = call <vilib>:"Pose3d_getRotation3d.vi"("in Pose3d"=w300) -> ("out Rotation3d"=w320:T2)  [unwired: 10 in]
  n164 = call <vilib>:"Pose3d_getXYZ.vi"("in Pose3d"=w300) -> ("Z"=w321:dbl, "Y"=w322:dbl, "X"=w323:dbl)  [unwired: 8 in]
  n165 = call <vilib>:"Util_ApproxEquals.vi"("Value 2"=w204, "Value 1"=w219) -> ("ApproxEquals"=w213:bool)  [unwired: 9 in]
  n166 = call <vilib>:"Util_ApproxEquals.vi"("Value 2"=w202, "Value 1"=w221) -> ("ApproxEquals"=w215:bool)  [unwired: 9 in]
  n167 = call <vilib>:"Util_ApproxEquals.vi"("Value 2"=w203, "Value 1"=w220) -> ("ApproxEquals"=w214:bool)  [unwired: 9 in]
  n168 = call <vilib>:"Rotation3d_GetXYZ.vi"("in Rotation3d"=w377) -> ("Z"=w374:dbl, "Y"=w375:dbl, "X"=w376:dbl)  [unwired: 8 in]
  n169 = for {
    tunnel: w4 -> [w435] mode=indexing
    tunnel: w3 -> [w432] mode=indexing
    shift-right: [w404] -> w1
    shift-left: TRUE -> [w405]
    w413 = 1e-05 ("Tolerance")
    n170 = call <vilib>:"Pose3d_Log.vi"("end Pose3d"=w432, "in Pose3d"=w435) -> ("out Twist3d"=w434:T9)  [unwired: 8 in, 1 out]
    n171 = call <vilib>:"Pose3d_Exp.vi"("Twist3d"=w434, "Pose3d"=w435) -> ("Updated Pose3d"=w433:T4)  [unwired: 8 in, 1 out]
    n172 = call <vilib>:"Pose3d_getRotation3d.vi"("in Pose3d"=w433) -> ("out Rotation3d"=w430:T2)  [unwired: 10 in]
    n173 = call <vilib>:"Pose3d_getRotation3d.vi"("in Pose3d"=w432) -> ("out Rotation3d"=w431:T2)  [unwired: 10 in]
    n174 = call <vilib>:"Pose3d_getXYZ.vi"("in Pose3d"=w433) -> ("Z"=w427:dbl, "Y"=w428:dbl, "X"=w429:dbl)  [unwired: 8 in]
    n175 = call <vilib>:"Pose3d_getXYZ.vi"("in Pose3d"=w432) -> ("Z"=w424:dbl, "Y"=w425:dbl, "X"=w426:dbl)  [unwired: 8 in]
    n176 = call <vilib>:"Rotation3d_GetQuaterion.vi"("in Rotation3d"=w430) -> ("out Quaterion"=w423:T3)  [unwired: 10 in]
    n177 = call <vilib>:"Rotation3d_GetQuaterion.vi"("in Rotation3d"=w431) -> ("out Quaterion"=w422:T3)  [unwired: 10 in]
    n178 = call <vilib>:"Quaternion_Get_All.vi"("Quaternion"=w422) -> ("Z"=w414:dbl, "Y"=w415:dbl, "X"=w416:dbl, "W"=w417:dbl)  [unwired: 7 in]
    n179 = call <vilib>:"Quaternion_Get_All.vi"("Quaternion"=w423) -> ("Z"=w418:dbl, "Y"=w419:dbl, "X"=w420:dbl, "W"=w421:dbl)  [unwired: 7 in]
    n180 = call <vilib>:"Util_ApproxEquals.vi"("Tolerance"=w413, "Value 2"=w426, "Value 1"=w429) -> ("ApproxEquals"=w412:bool)  [unwired: 8 in]
    n181 = call <vilib>:"Util_ApproxEquals.vi"("Tolerance"=w413, "Value 2"=w425, "Value 1"=w428) -> ("ApproxEquals"=w411:bool)  [unwired: 8 in]
    n182 = call <vilib>:"Util_ApproxEquals.vi"("Tolerance"=w413, "Value 2"=w424, "Value 1"=w427) -> ("ApproxEquals"=w410:bool)  [unwired: 8 in]
    n183 = call <vilib>:"Util_ApproxEquals.vi"("Tolerance"=w413, "Value 2"=w417, "Value 1"=w421) -> ("ApproxEquals"=w409:bool)  [unwired: 8 in]
    n184 = call <vilib>:"Util_ApproxEquals.vi"("Tolerance"=w413, "Value 2"=w415, "Value 1"=w419) -> ("ApproxEquals"=w407:bool)  [unwired: 8 in]
    n185 = call <vilib>:"Util_ApproxEquals.vi"("Tolerance"=w413, "Value 2"=w416, "Value 1"=w420) -> ("ApproxEquals"=w408:bool)  [unwired: 8 in]
    n186 = call <vilib>:"Util_ApproxEquals.vi"("Tolerance"=w413, "Value 2"=w414, "Value 1"=w418) -> ("ApproxEquals"=w406:bool)  [unwired: 8 in]
    n187 = Compound Arithmetic op=OR(w412, w411, w410, w409, w408, w407, w406, w405) -> (w404:bool)
  }
  "Exp/Log \nTest Passed" <- w1
  n188 = call <vilib>:"Rotation3d_GetXYZ.vi"("in Rotation3d"=w320) -> ("Z"=w317:dbl, "Y"=w318:dbl, "X"=w319:dbl)  [unwired: 8 in]
  n189 = call <vilib>:"Util_ApproxEquals.vi"("Value 2"=w123, "Value 1"=w124) -> ("ApproxEquals"=w118:bool)  [unwired: 9 in]
  n190 = call <vilib>:"Util_ApproxEquals.vi"("Value 2"=w121, "Value 1"=w122) -> ("ApproxEquals"=w117:bool)  [unwired: 9 in]
  n191 = call <vilib>:"Util_ApproxEquals.vi"("Value 2"=w119, "Value 1"=w120) -> ("ApproxEquals"=w116:bool)  [unwired: 9 in]
  n192 = call <vilib>:"Util_ApproxEquals.vi"("Value 2"=0.0, "Value 1"=w378) -> ("ApproxEquals"=w371:bool)  [unwired: 9 in]
  n193 = call <vilib>:"Util_ApproxEquals.vi"("Value 2"=w361, "Value 1"=w380) -> ("ApproxEquals"=w373:bool)  [unwired: 9 in]
  n194 = call <vilib>:"Util_ApproxEquals.vi"("Value 2"=w360, "Value 1"=w379) -> ("ApproxEquals"=w372:bool)  [unwired: 9 in]
  n195 = call <vilib>:"Util_ApproxEquals.vi"("Value 2"=0.0, "Value 1"=w321) -> ("ApproxEquals"=w314:bool)  [unwired: 9 in]
  n196 = call <vilib>:"Util_ApproxEquals.vi"("Value 2"=w299, "Value 1"=w323) -> ("ApproxEquals"=w316:bool)  [unwired: 9 in]
  n197 = call <vilib>:"Util_ApproxEquals.vi"("Value 2"=0.0, "Value 1"=w322) -> ("ApproxEquals"=w315:bool)  [unwired: 9 in]
  n198 = call <vilib>:"Util_ApproxEquals.vi"("Value 2"=w352, "Value 1"=w374) -> ("ApproxEquals"=w368:bool)  [unwired: 9 in]
  n199 = call <vilib>:"Util_ApproxEquals.vi"("Value 2"=w350, "Value 1"=w376) -> ("ApproxEquals"=w370:bool)  [unwired: 9 in]
  n200 = call <vilib>:"Util_ApproxEquals.vi"("Value 2"=w351, "Value 1"=w375) -> ("ApproxEquals"=w369:bool)  [unwired: 9 in]
  n201 = call <vilib>:"Util_ApproxEquals.vi"("Value 2"=w303, "Value 1"=w317) -> ("ApproxEquals"=w311:bool)  [unwired: 9 in]
  n202 = call <vilib>:"Util_ApproxEquals.vi"("Value 2"=w301, "Value 1"=w319) -> ("ApproxEquals"=w313:bool)  [unwired: 9 in]
  n203 = call <vilib>:"Util_ApproxEquals.vi"("Value 2"=w302, "Value 1"=w318) -> ("ApproxEquals"=w312:bool)  [unwired: 9 in]
  n204 = Compound Arithmetic op=AND(w218, w217, w216, w215, w214, w213) -> (w200:bool)
  n205 = Compound Arithmetic op=AND(w118, w117, w116) -> (w115:bool)
  n206 = Compound Arithmetic op=AND(w373, w372, w371, w370, w369, w368) -> (w348:bool)
  n207 = Compound Arithmetic op=AND(w316, w315, w314, w313, w312, w311) -> (w297:bool)
  n208 = Compound Arithmetic op=AND(w348, w297, w272, w246, w200, w177, w115, w1) -> (→"All PASSED":bool)
  "error out" <- "error in (no error)"
